vi "Setup DAQ.vi"(8 "error in":errorcluster, 11 "Cluster":T1={"physical channel"="cDAQ9181-1913300Mod1/ai0", "minimum value"=0.0, "maximum value"=94400.0, "number of samples"=10, "rate"=125.0, "custom scale name"="Pressure"}) -> (0 "error out":errorcluster, 3 "task out":refnum<k21>)   [LabVIEW 2025]
uses:
  Libraries/Settings Editor/DAQ Settings.ctl
  <vilib>/DAQmx/create/channels.llb/DAQmx Create Channel (AI-Current-Basic).vi
  <vilib>/DAQmx/configure/timing.llb/DAQmx Timing (Sample Clock).vi
  <resource>/objmgr/daqmx.rc
panel:
  out "AI.Filter.Order":u32
  out "AI.Filter.Response":i32(ring)=16152 items=["Comb"=16152, "Bessel"=16153, "Brickwall"=16155, "Butterworth"=16076]
  out "AI.Filter.Freq":dbl
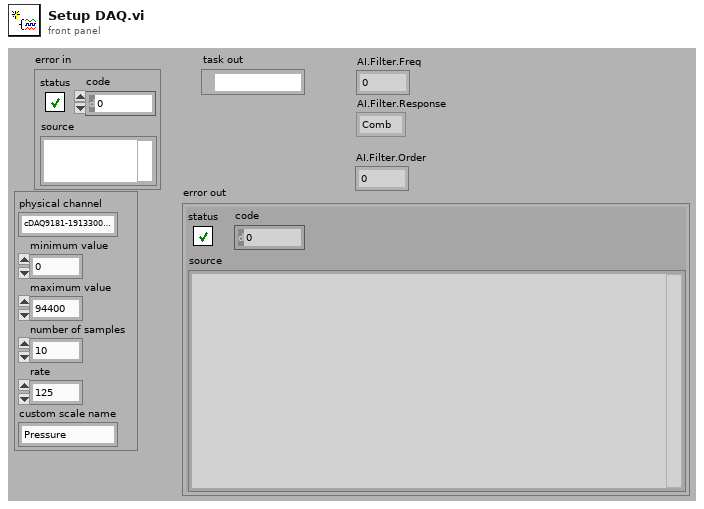
[diagram p1: front panel]
types:
  T1 = typedef "DAQ Settings.ctl" = cluster{"physical channel":string, "minimum value":dbl, "maximum value":dbl, "number of samples":i32, "rate":dbl, "custom scale name":string}
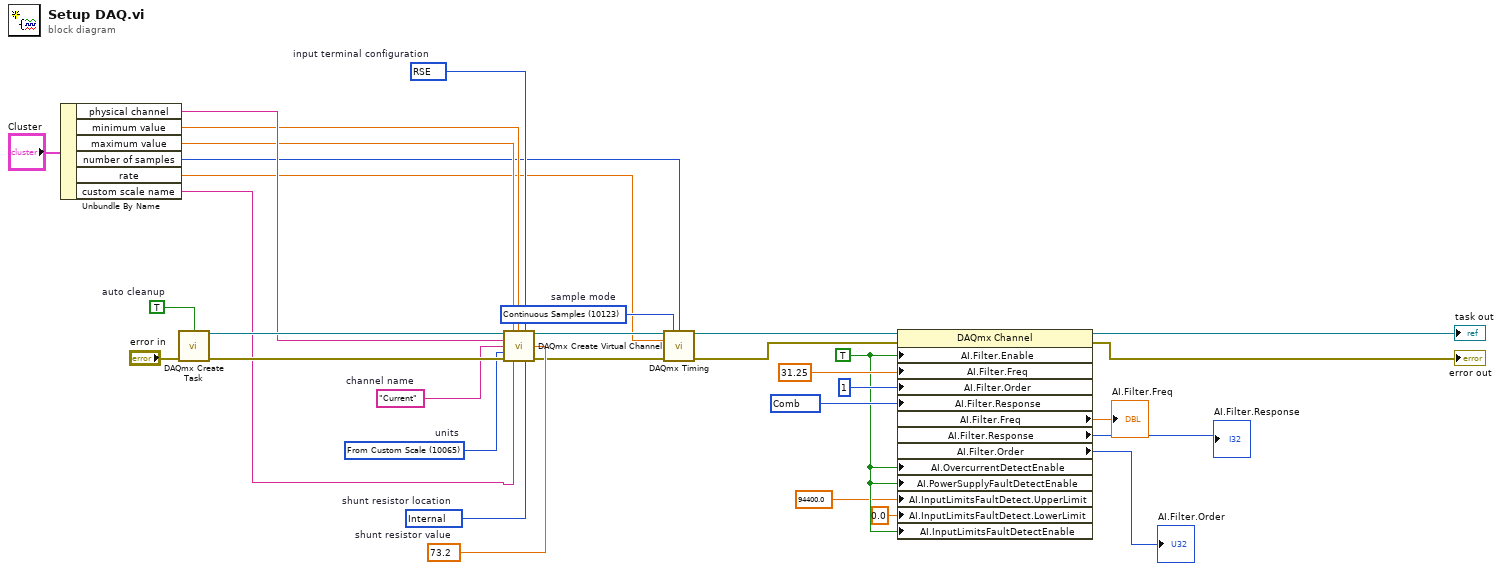
[diagram p0: block diagram]
diagram:
  w16 = 16152 items=["Comb"=16152, "Bessel"=16153, "Brickwall"=16155, "Butterworth"=16076] ("AI.Filter.Response")
  w10 = TRUE ("AI.Filter.Enable")
  w23 = 10123 items=["Finite Samples"=10178, "Continuous Samples"=10123, "Hardware Timed Single Point"=12522]  # sample mode
  w24 = 10083 items=["default"=-1, "RSE"=10083, "NRSE"=10078, "Differential"=10106, "Pseudodifferential"=12529]  # input terminal configuration
  w25 = 10065 items=["Amps"=10342, "From Custom Scale"=10065]  # units
  w26 = 73.2  # shunt resistor value
  w27 = 10200 items=["Internal"=10200, "External"=10167]  # shunt resistor location
  w28 = "Current"  # channel name
  w30 = TRUE  # auto cleanup
  n1 = Unbundle By Name("Cluster") -> ("physical channel"=w6:string, "minimum value"=w5:dbl, "maximum value"=w4:dbl, "number of samples"=w3:i32, "rate"=w2:dbl, "custom scale name"=w1:string)
  n2 = call <vilib>:"DAQmx Create Task.vi"("auto cleanup"=w30, "error in"="error in") -> ("task out"=w29:refnum<k21>, "error out"=w31:errorcluster)  [unwired: 12 in]
  n3 = call-poly <vilib>:"DAQmx Create Virtual Channel.vi"("task in"=w29, "maximum value"=w4, "minimum value"=w5, "input terminal configuration"=w24, "physical channels"=w6, "name to assign"=w28, "external shunt resistor value"=w26, "units"=w25, "error in"=w31, "custom scale name"=w1, "shunt resistor location"=w27) -> ("task out"=w17:refnum<k21>, "error out"=w18:errorcluster)  [unwired: 3 in]
  n4 = call-poly <vilib>:"DAQmx Timing.vi"("task/channels in"=w17, "sample mode"=w23, "samples per channel"=w3, "rate"=w2, "error in"=w18) -> ("task out"=w20:refnum<k21>, "error out"=w19:errorcluster)  [unwired: 9 in]
  n5 = property class="DAQmx Channel"(reference=w20, error in=w19, "AI.Filter.Enable"=w10, "AI.Filter.Freq"=31.25, "AI.Filter.Order"=u32 1, "AI.Filter.Response"=w16, "AI.OvercurrentDetectEnable"=w10, "AI.PowerSupplyFaultDetectEnable"=w10, "AI.InputLimitsFaultDetect.UpperLimit"=94400.0, "AI.InputLimitsFaultDetect.LowerLimit"=0.0, "AI.InputLimitsFaultDetectEnable"=w10) -> (reference out=→"task out":refnum<k21>, error out=→"error out":errorcluster, "AI.Filter.Freq"=→"AI.Filter.Freq":dbl, "AI.Filter.Response"=→"AI.Filter.Response":i32, "AI.Filter.Order"=→"AI.Filter.Order":u32)
